vi "Bus0_Dev1_Ch2.vi"(7 "FIFOs: I/O Node":T1={"SendCmdFIFO"="Bus0_Dev1_Ch2_Tx_FIFO", "ReceiveDataFIFO"="Bus0_Dev1_Ch2_Rx_FIFO"}) -> (8 "Received Data":u64)   [LabVIEW 2014]
uses:
  Node/Controls/Node_Command_Sent.ctl
  Node/Controls/NodeResources FIFOs.ctl
  <vilib>/Platform/TimedLoop/XDataNode/timing_clust.ctl
  <vilib>/Platform/TimedLoop/XDataNode/nitl_modes.ctl
  <vilib>/Platform/TimedLoop/XDataNode/wakeup.ctl
  <vilib>/Platform/TimedLoop/XDataNode/XDataNode.xnode
  IO Node Logic Template_SPIBus0.lvlib
  <vilib>/Platform/TimedLoop/XDataNode/XDNodeRunTimeDep.lvlib
panel:
  in  "Command":T2={"Device ID"=1, "Data"=0, "Command"=0, "Node ID"=4, "Misc"=0}
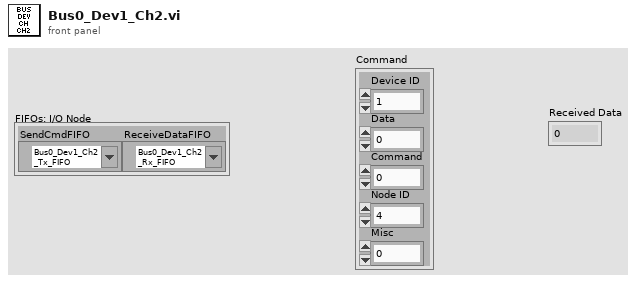
[diagram p1: front panel]
types:
  T1 = typedef "IO Node Logic Template_SPIBus0.lvlib/NodeResources FIFOs.ctl" = cluster{"SendCmdFIFO":refnum<k21>, "ReceiveDataFIFO":refnum<k21>}
  T2 = typedef "IO Node Logic Template_SPIBus0.lvlib/Node_Command_Sent.ctl" = cluster{"Device ID":u8, "Data":u64, "Command":u8, "Node ID":u8, "Misc":u8}
  T3 = typedef "XDNodeRunTimeDep.lvlib/timing_clust.ctl" = cluster{"Expected End [f-1]":u64, "Actual End [f-1]":u64, "Finished Late? [f-1]":bool, "Expected End [i-1]":u64, "Actual End [i-1]":u64, "Finished Late? [i-1]":bool, "Expected Start [i]":u64, "Actual Start [i]":u64, "Expected Start [f]":u64, "Actual Start [f]":u64, "Source Name":string, "Structure Name":string, "Period":i64, "Deadline":i64, "Offset":i64, "Start":i64, "Priority":i32, "Timeout":i32, "Mode":T4, "Wakeup Reason":T5, "Error":errorcluster, "Source Type":string, "Secondary Source Type":string, "Global End Time":u64, "Global Start Time":u64, "Frame Duration":u64, "Iteration Duration":u64, "Assigned CPU":i32, "I/O Scan Engine Mode":u32}
  T4 = typedef "XDNodeRunTimeDep.lvlib/nitl_modes.ctl" = enum32{"No Change", "Process missed periods, maintain original phase", "Discard missed periods, maintain original phase", "Process missed periods, ignore original phase", "Discard missed periods, ignore original phase"}
  T5 = typedef "XDNodeRunTimeDep.lvlib/wakeup.ctl" = enum32{"Normal", "Aborted", "Asynchronous wakeup", "Timing source error", "Timed loop error", "Timeout"}
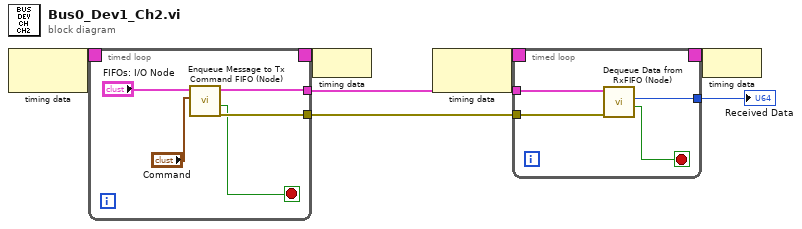
[diagram p0: block diagram]
diagram:
  n1 = node-c288() -> (w4:T3)  [unwired: 1 in]
  n2 = timed-loop {
    timing: w4 -> [_]
    timing-out: [_] -> w3
    tunnel: [w12] -> w7
    tunnel: [w11] -> w6
    stop <- w10 stop-if-true
    n3 = call "Enqueue Message to Tx Command FIFO (Node).vi"("Command"="Command", "FIFOs: I/O Node"="FIFOs: I/O Node") -> ("error out"=w12:errorcluster, "Success?"=w10:bool, "FIFOs: I/O Node"=w11:T1)  [unwired: 7 in]
  }
  n4 = node-c288(w3) -> ()
  n5 = node-c288() -> (w2:T3)  [unwired: 1 in]
  n6 = timed-loop {
    timing: w2 -> [_]
    timing-out: [_] -> w1
    tunnel: w7 -> [w18]
    tunnel: w6 -> [w17]
    tunnel: [w16] -> w5
    stop <- w15 stop-if-true
    n7 = call "Dequeue Data from RxFIFO (Node).vi"("error in"=w18, "FIFOs: I/O Node"=w17) -> ("Received Data Valid"=w15:bool, "Received Data"=w16:u64)  [unwired: 6 in, 2 out]
  }
  "Received Data" <- w5
  n8 = node-c288(w1) -> ()
